vi "Get Line Timing.vi"(8 "error in (no error)":errorcluster, 10 "Line index":i32, 11 "Pulseblaster in":refnum<class "Pulseblaster.lvclass">) -> (0 "error out":errorcluster, 1 "parsed t":dbl, 2 "n steps":i32, 3 "Pulseblaster out":refnum<class "Pulseblaster.lvclass">, 4 "Mode":string, 5 "parsed dt":dbl, 7 "Group enabled?":bool)   [LabVIEW 2013, in "Pulseblaster.lvclass"]
doc: "Parse all master timing information for a specific table line."
uses:
  Pulseblaster.lvclass
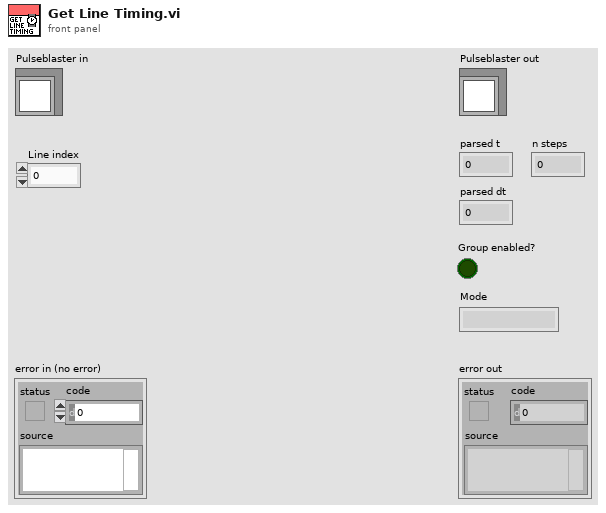
[diagram p1: front panel]
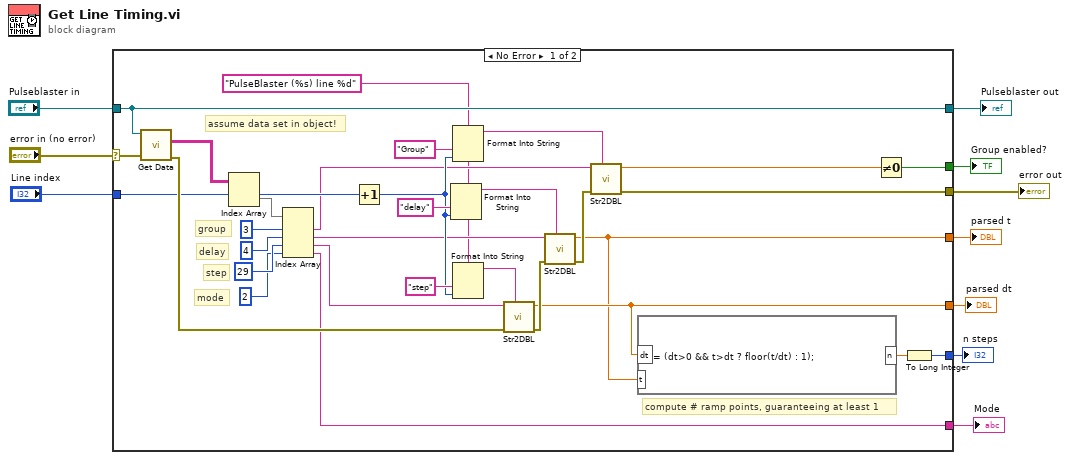
[diagram p0: block diagram]
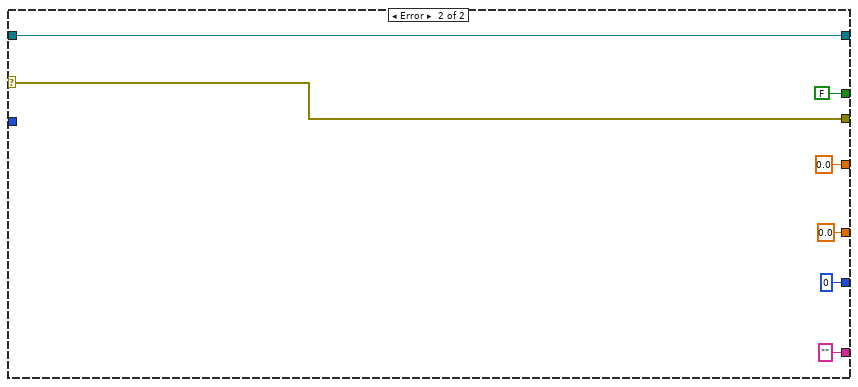
[diagram p2: hidden frame]
diagram:
  n1 = case shown="No Error" "error in (no error)" {
    selector: "error in (no error)" -> [w40 w48]
    tunnel: [w26 w48] -> w4
    tunnel: [w41 w47] -> w3
    tunnel: "Pulseblaster in" -> [w41 w47]
    tunnel: [w12 0.0 ("delay")] -> w7
    tunnel: [w13 0.0 ("dt")] -> w6
    tunnel: [w33 FALSE ("Group enabled?")] -> w5
    tunnel: "Line index" -> [w22 _]
    tunnel: [w16 ""] -> w2
    tunnel: [w11 0] -> w1
    frame No Error {
      w15 = "PulseBlaster (%s) line %d"
      # "compute # ramp points, guaranteeing at least 1"
      # "assume data set in object!"
      # "mode"
      # "step"
      # "delay"
      # "group"
      n2 = call-dynamic "Get Data.vi"("error in (no error)"=w40, "Device in"=w41) -> ("error out"=w27:errorcluster, "Table Indicator"=w39:string[][])  [unwired: 6 in, 1 out]
      n3 = Index Array(array=w39, index (row)=w22) -> (element=w38:string[])  [unwired: 1 in]
      n4 = Index Array(array=w38, index #1=3 ("index"), index #2=4 ("index"), index #3=29 ("index"), index #4=2 ("index")) -> (element #1=w18:string, element #2=w19:string, element #3=w20:string, element #4=w16:string)
      n5 = Increment(x=w22) -> (x+1=w21:i32)
      n6 = Format Into String(format string=w15, "delay" ("input 1"), w21) -> (resulting string=w31:string)  [unwired: 2 in, 1 out]
      n7 = Format Into String(format string=w15, "Group" ("input 1"), w21) -> (resulting string=w32:string)  [unwired: 2 in, 1 out]
      n8 = Format Into String(format string=w15, "step" ("input 1"), w21) -> (resulting string=w30:string)  [unwired: 2 in, 1 out]
      n9 = call "Str2DBL.vi"("Error Locator"=w30, "error in (no error)"=w27, "formula"=w20) -> ("error out"=w29:errorcluster, "y value"=w13:dbl)  [unwired: 5 in]
      n10 = call "Str2DBL.vi"("Error Locator"=w31, "error in (no error)"=w29, "formula"=w19) -> ("error out"=w28:errorcluster, "y value"=w12:dbl)  [unwired: 5 in]
      n11 = call "Str2DBL.vi"("Error Locator"=w32, "error in (no error)"=w28, "formula"=w18) -> ("error out"=w26:errorcluster, "y value"=w34:dbl)  [unwired: 5 in]
      n12 = formula code="n= (dt>0 && t>dt ? floor(t/dt) : 1);"("dt"=w13, "t"=w12) -> ("n"=w14:dbl)
      n13 = Not Equal To 0?(x=w34) -> (x != 0?=w33:bool)
      n14 = To Long Integer(number=w14) -> (32bit integer=w11:i32)
    }
    frame Error {
    }
  }
  "error out" <- w4
  "Pulseblaster out" <- w3
  "parsed t" <- w7
  "parsed dt" <- w6
  "Group enabled?" <- w5
  "Mode" <- w2
  "n steps" <- w1
